vi "Translate to Array Data_3.vi"(0 "original data":path=path "C:/Users/User/Desktop/aaa.csv", 1 "Only Use Last Value?":bool=TRUE, 2 "Electrode number, N":u16=8, 3 "Current Mode":u8[][](array[numeric]), 5 "original error":errorcluster, 7 "Array Mode":u16(ring) items=["None", "Gradient + Dipole dipole", "Gradient", "Dipole Dipole", "Schlumberger"], 9 "modified data":path=path "C:/Users/User/Desktop/test.csv", 11 "modified error":errorcluster, 12 "Inverse\nPolarity":bool=TRUE, 13 "Insert\nBreak":bool=TRUE, 14 "External\nRef":bool=TRUE) -> (4 "original data path":path, 6 "original data error out":errorcluster)   [LabVIEW 2023]
uses:
  <vilib>/Utility/error.llb/DialogType.ctl
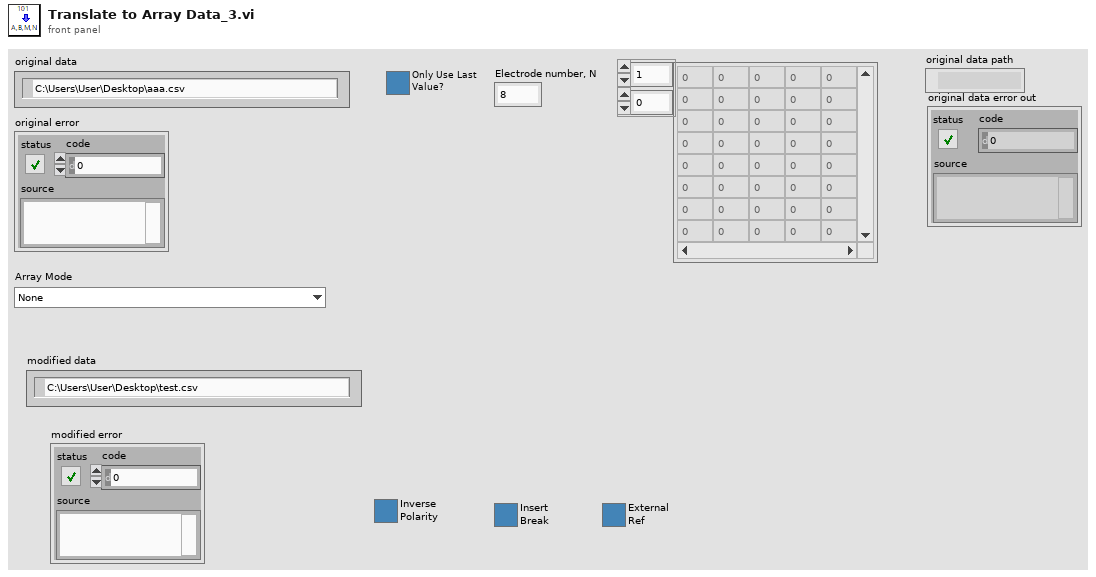
[diagram p1: front panel]
types:
  T1 = enum16{"open", "replace", "create", "open or create", "replace or create", "replace or create with confirmation"}
  T2 = typedef "DialogType.ctl" = u16
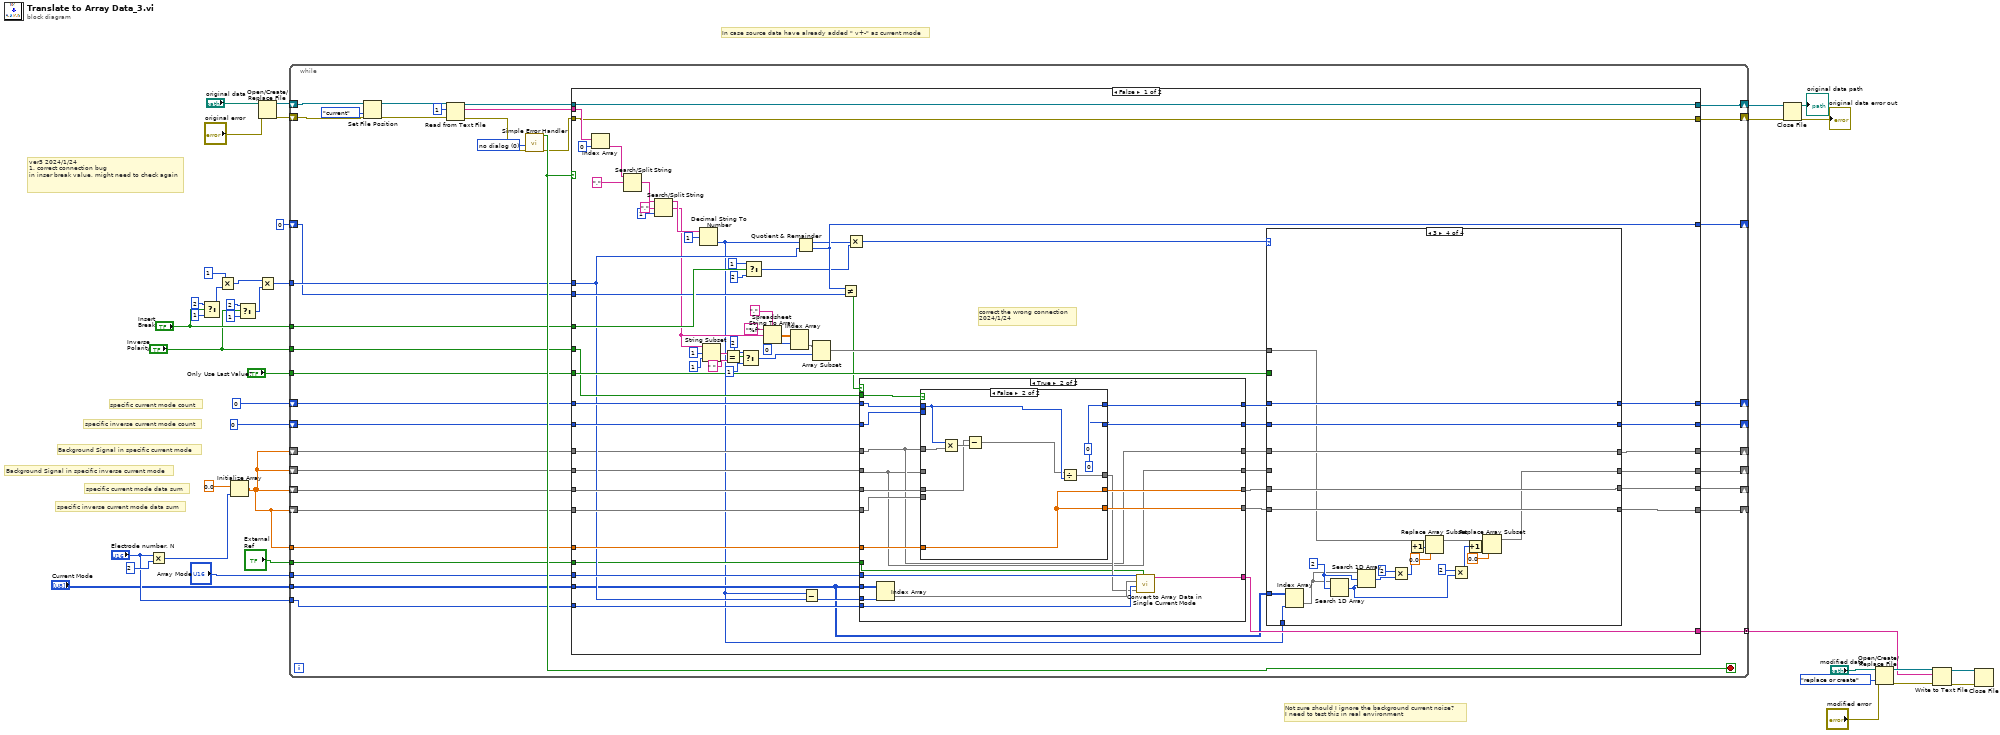
[diagram p0: block diagram]
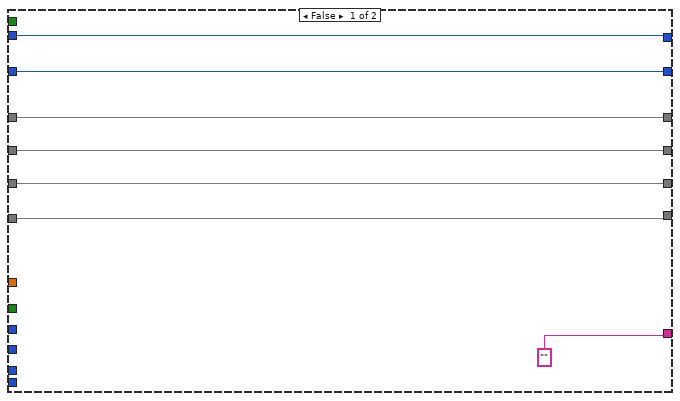
[diagram p2: hidden frame]
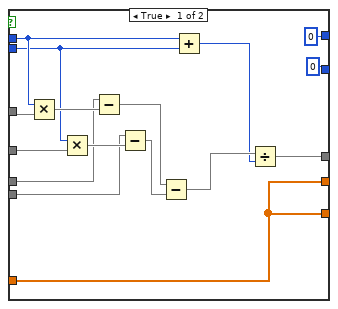
[diagram p3: hidden frame]
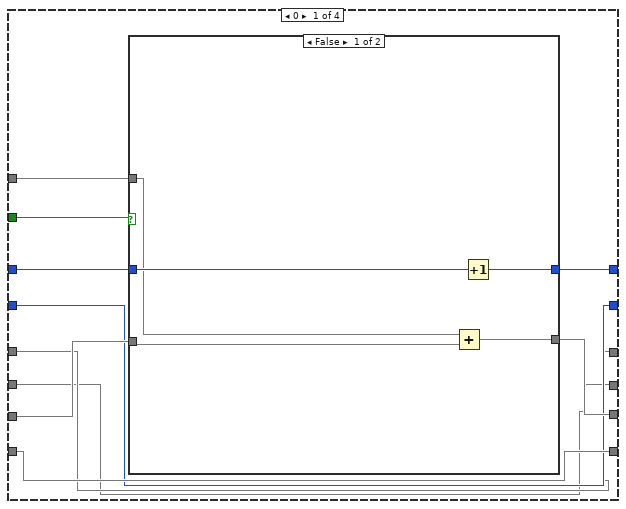
[diagram p4: hidden frame]
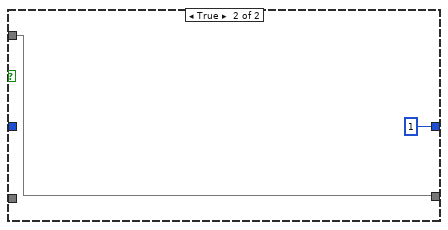
[diagram p5: hidden frame]
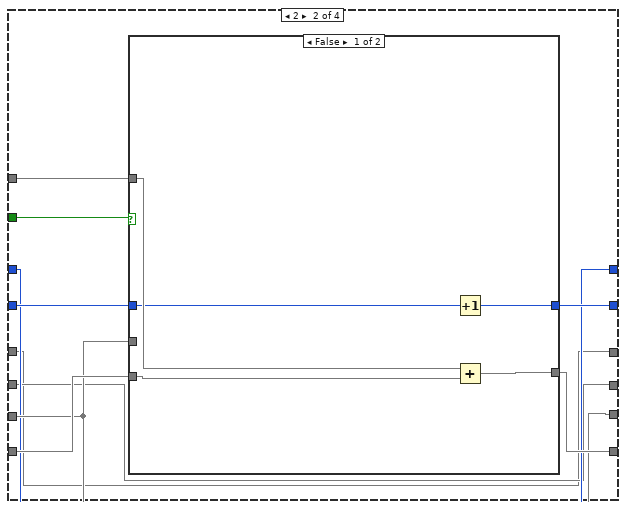
[diagram p6: hidden frame]
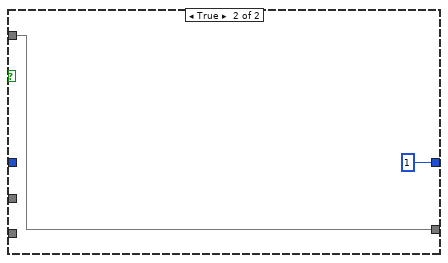
[diagram p7: hidden frame]
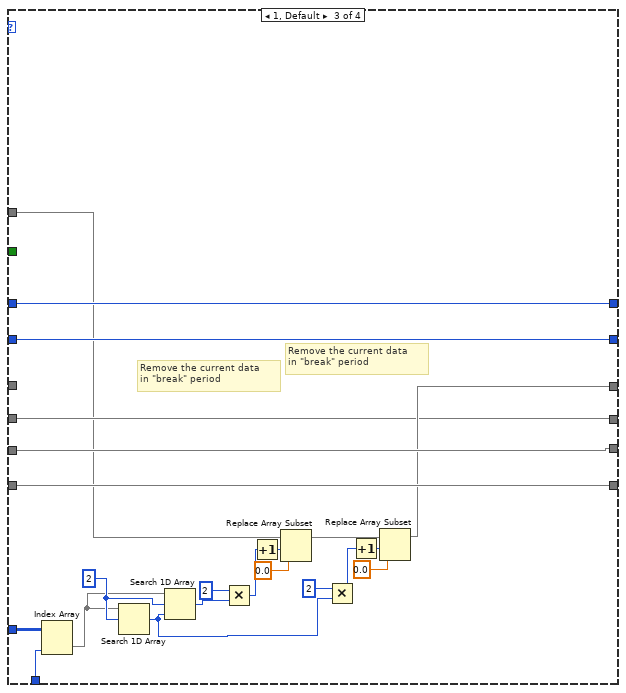
[diagram p8: hidden frame]
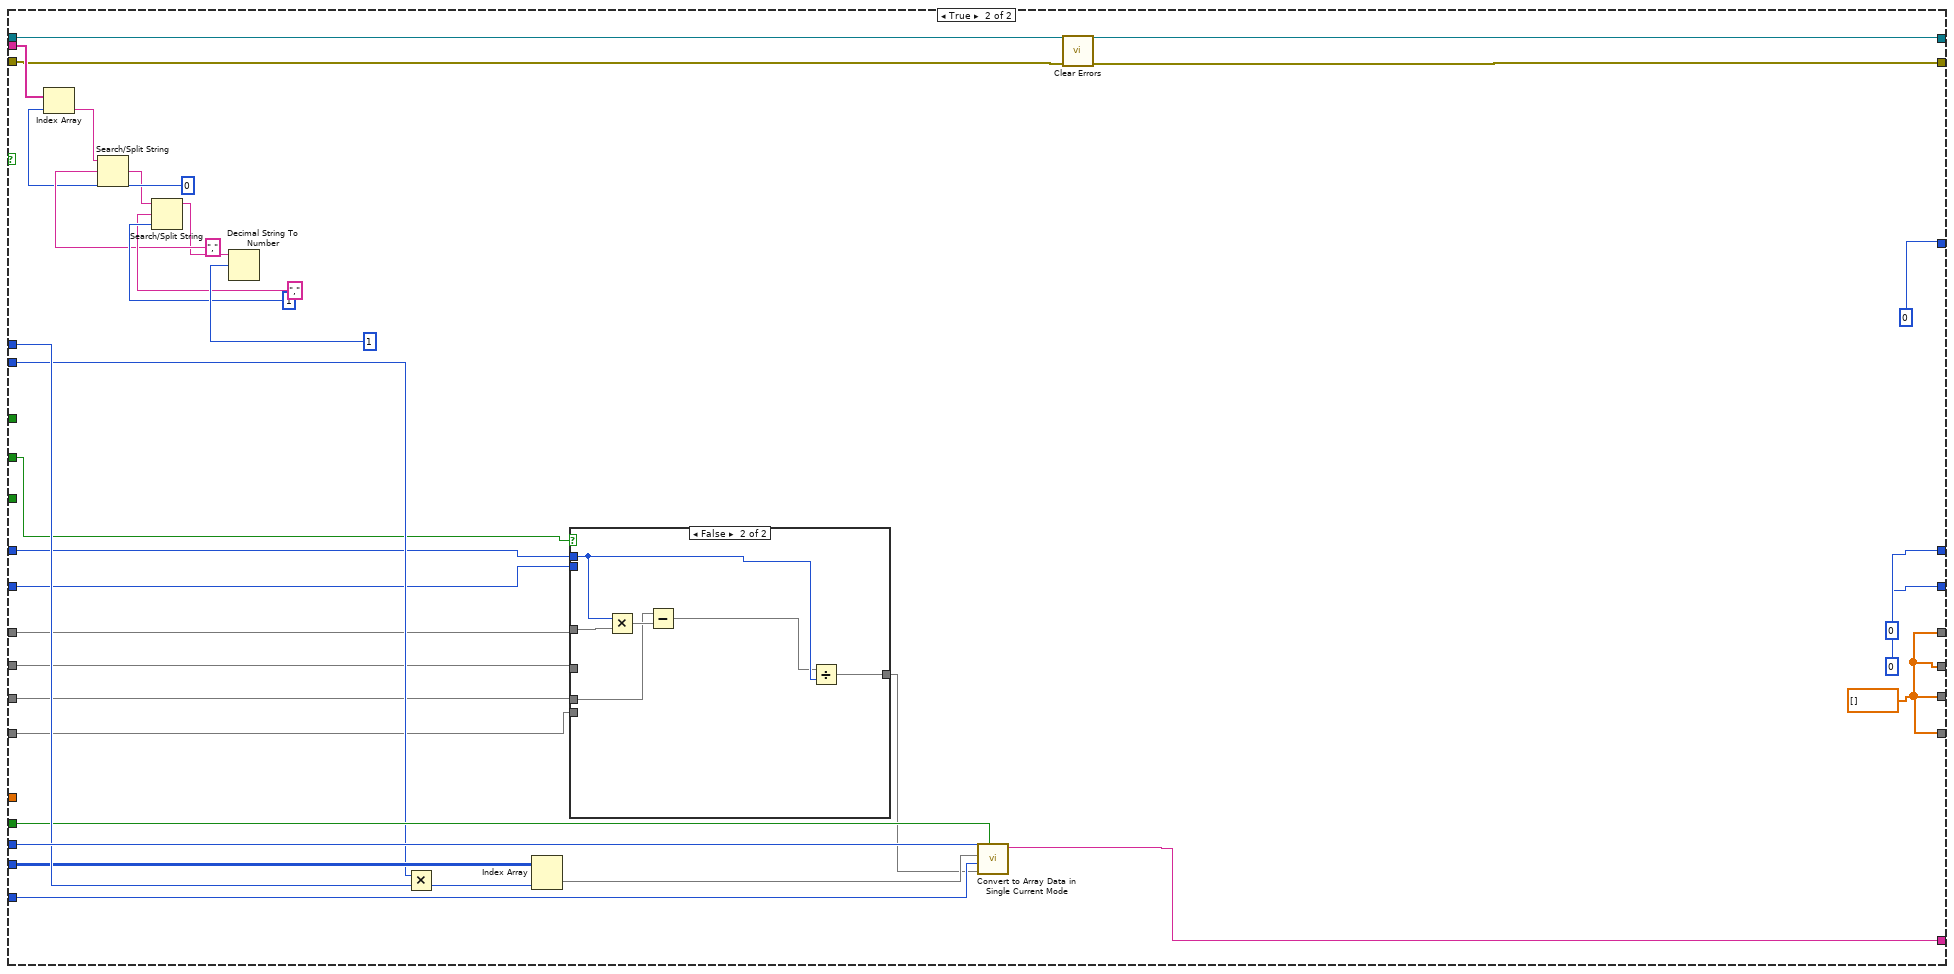
[diagram p9: hidden frame]
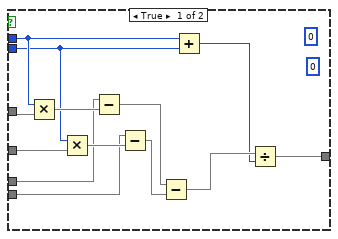
[diagram p10: hidden frame]
diagram:
  # "Not sure should I ignore the background current noise?\nI need to test this in real environment"
  # "ver3 2024/1/24\n1. correct connection bug\nin inser break value, might need to check again"
  # "Background Signal in specific inverse current mode"
  # "Background Signal in specific current mode"
  # "In case source data have already added \" v+-\" as current mode"
  # "specific inverse current mode data sum"
  # "specific current mode data sum"
  # "specific inverse current mode count"
  # "specific current mode count"
  n1 = Multiply(x="Electrode number, N", y=u16 2) -> (x*y=w13:u16)
  n2 = Select(t=2 ("number"), s="Insert\nBreak", f=1 ("number")) -> (s? t:f=w22:i32)
  n3 = Multiply(x=1 ("number"), y=w22) -> (x*y=w16:i32)
  n4 = Initialize Array(0.0 ("element"), w13) -> (w3:dbl[])
  n5 = Select(t=2 ("number"), s="Inverse\nPolarity", f=1 ("number")) -> (s? t:f=w21:i32)
  n6 = Open/Create/Replace File(file path (use dialog)="original data", error in="original error") -> (refnum out=w36:refnum<file>, error out=w37:errorcluster)  [unwired: 4 in, 1 out]
  n7 = Multiply(x=w16, y=w21) -> (x*y=w20:i32)
  n8 = while {
    shift-right: [w69] -> w31
    shift-left: w37 -> [w76]
    shift-right: [w68] -> w38
    shift-left: w36 -> [w67]
    tunnel: "Insert\nBreak" -> [w63]
    tunnel: "Inverse\nPolarity" -> [w62]
    tunnel: "Only Use Last Value?" -> [w61]
    tunnel: w20 -> [w60]
    shift-right: [w55] -> _
    shift-left: 0 ("number") -> [w59]
    shift-right: [w52] -> _
    shift-left: 0 ("number") -> [w58]
    shift-right: [w54] -> _
    shift-left: w3 -> [w57]
    shift-right: [w53] -> _
    shift-left: w3 -> [w56]
    shift-right: [w51] -> _
    shift-left: 0 -> [w50]
    tunnel: w3 -> [w49]
    tunnel: "Current Mode" -> [w47]
    tunnel: "Array Mode" -> [w48]
    tunnel: "Electrode number, N" -> [w46]
    tunnel: "External\nRef" -> [w45]
    tunnel: [w44] -> w7 mode=concatenating
    shift-right: [w41] -> _
    shift-left: w3 -> [w43]
    shift-right: [w40] -> _
    shift-left: w3 -> [w42]
    stop <- w73 stop-if-true
    w74 = T2 0 items=["no dialog", "OK message", "continue or stop message", "OK message + warnings", "continue/stop + warnings"] ("type of dialog (OK msg:1)")
    n9 = Set File Position(refnum=w67, from (0:start)=enum16{"start", "end", "current"}."current", error in=w76) -> (refnum out=w66:refnum<file>, error out=w65:errorcluster)  [unwired: 1 in]
    n10 = Read from Text File(file (use dialog)=w66, count=1, error in=w65) -> (refnum out=w71:refnum<file>, text=w72:string[], error out=w70:errorcluster)  [unwired: 1 in, 1 out]
    n11 = call <vilib>:"Simple Error Handler.vi"("type of dialog (OK msg:1)"=w74, "error in (no error)"=w70) -> ("error?"=w73:bool, "error out"=w64:errorcluster)  [unwired: 3 in, 3 out]
    n12 = case shown="False" w73 {
      tunnel: w72 -> [w137 w300]
      tunnel: w71 -> [w134 w297]
      tunnel: w64 -> [w133 w285]
      tunnel: [w134 w297] -> w68
      tunnel: [w133 w284] -> w69
      tunnel: w63 -> [w130 _]
      tunnel: w62 -> [w110 w275]
      tunnel: w61 -> [w129 _]
      tunnel: w60 -> [w98 w292]
      tunnel: w59 -> [w114 w274]
      tunnel: w58 -> [w113 w273]
      tunnel: w57 -> [w112 w278]
      tunnel: w56 -> [w111 w279]
      tunnel: [w120 0 ("number")] -> w55
      tunnel: [w119 w280] -> w54
      tunnel: [w118 w280] -> w53
      tunnel: [w117 0 ("number")] -> w52
      tunnel: [w115 0] -> w51
      tunnel: w50 -> [w116 w281]
      tunnel: w49 -> [w104 _]
      tunnel: w48 -> [w100 w294]
      tunnel: w47 -> [w81 w282]
      tunnel: w46 -> [w97 w291]
      tunnel: w45 -> [w96 w290]
      tunnel: [w95 w289] -> w44
      tunnel: w43 -> [w85 w276]
      tunnel: w42 -> [w84 w277]
      tunnel: [w79 w280] -> w41
      tunnel: [w78 w280] -> w40
      frame False {
        # "correct the wrong connection\n2024/1/24"
        n13 = Index Array(array=w137, index=0) -> (element=w135:string)
        n14 = Search/Split String(string=w135, search string/char (-)=",") -> (match + rest of string=w125:string)  [unwired: 1 in, 2 out]
        n15 = Search/Split String(string=w125, search string/char (-)=",", offset (0)=1) -> (substring before match=w126:string, match + rest of string=w87:string)  [unwired: 1 out]
        n16 = Decimal String To Number(string=w126, offset=1) -> (number=w80:i32)  [unwired: 1 in, 1 out]
        n17 = String Subset(string=w87, offset (0)=1, length (rest)=1 ("length (rest)")) -> (substring=w94:string)
        n18 = Equal?(x=w94, y=" ") -> (x = y?=w93:bool)
        n19 = Select(t=2 ("index (row)"), s=w93, f=1 ("index (row)")) -> (s? t:f=w86:i32)
        n20 = Select(t=1, s=w130, f=2 ("y")) -> (s? t:f=w103:i32)
        n21 = Spreadsheet String To Array(delimiter (Tab)=",", format string="%f", spreadsheet string=w87) -> (array=w124:dbl[][])  [unwired: 1 in]
        n22 = Index Array(array=w124, index (row)=0) -> (element=w122:dbl[])  [unwired: 1 in]
        n23 = Quotient & Remainder(x=w80, y=w98) -> (x-y*floor(x/y)=w102:i32, floor(x/y)=w115:i32)
        n24 = Subtract(x=w80, y=w98) -> (x-y=w99:i32)
        n25 = Array Subset(array=w122, index=w86) -> (w121:dbl[])  [unwired: 1 in]
        n26 = Not Equal?(x=w115, y=w116) -> (x != y?=w105:bool)
        n27 = Multiply(x=w102, y=w103) -> (x*y=w101:i32)
        n28 = case shown="True" w105 {
          tunnel: w114 -> [w148 w165]
          tunnel: w113 -> [w147 w164]
          tunnel: w112 -> [w146 w167]
          tunnel: w111 -> [w145 w166]
          tunnel: w110 -> [_ w168]
          tunnel: [w148 w163] -> w109
          tunnel: [w147 w162] -> w108
          tunnel: [w146 w161] -> w107
          tunnel: [w145 w160] -> w106
          tunnel: w104 -> [_ w159]
          tunnel: w100 -> [_ w155]
          tunnel: w81 -> [_ w158]
          tunnel: w99 -> [_ w157]
          tunnel: w97 -> [_ w154]
          tunnel: w96 -> [_ w152]
          tunnel: ["" ("String") w151] -> w95
          tunnel: w85 -> [w143 w150]
          tunnel: w84 -> [w142 w149]
          tunnel: [w143 w150] -> w83
          tunnel: [w142 w149] -> w82
          frame False {
          }
          frame True {
            n29 = Index Array(array=w158, index (col)=w157) -> (element=w156:u8[])  [unwired: 1 in]
            n30 = case shown="False" w168 {
              tunnel: w167 -> [w173 w186]
              tunnel: w166 -> [w172 _]
              tunnel: w165 -> [w174 w188]
              tunnel: w164 -> [w169 _]
              tunnel: [0 ("number") 0 ("number")] -> w163
              tunnel: [0 ("number") 0 ("number")] -> w162
              tunnel: [w180 w191] -> w161
              tunnel: [w180 w191] -> w160
              tunnel: w159 -> [w180 w191]
              tunnel: [w179 w190] -> w153
              tunnel: w150 -> [w177 w189]
              tunnel: w149 -> [w175 _]
              frame True {
                n31 = Multiply(x=w174, y=w177) -> (x*y=w178:dbl[])
                n32 = Multiply(x=w169, y=w175) -> (x*y=w176:dbl[])
                n33 = Subtract(x=w173, y=w178) -> (x-y=w170:dbl[])
                n34 = Subtract(x=w172, y=w176) -> (x-y=w171:dbl[])
                n35 = Subtract(x=w170, y=w171) -> (x-y=w184:dbl[])
                n36 = Add(x=w174, y=w169) -> (x+y=w183:i32)
                n37 = Divide(x=w184, y=w183) -> (x/y=w179:dbl[])
              }
              frame False {
                n38 = Multiply(x=w188, y=w189) -> (x*y=w187:dbl[])
                n39 = Subtract(x=w186, y=w187) -> (x-y=w185:dbl[])
                n40 = Divide(x=w185, y=w188) -> (x/y=w190:dbl[])
              }
            }
            n41 = call "Convert to Array Data in Single Current Mode.vi"("External\nRef"=w152, "data"=w153, "Electrode number, N"=w154, "Current Mode"=w156, "Array Mode"=w155) -> ("String"=w151:string)  [unwired: 6 in]
          }
        }
        n42 = case shown="3" w101 {
          tunnel: w129 -> [w203 w220 _ _]
          tunnel: w121 -> [w199 w219 w228 w250]
          tunnel: w109 -> [w202 w213 w249 w271]
          tunnel: w108 -> [w196 w216 w248 w270]
          tunnel: w107 -> [w201 w214 w247 w269]
          tunnel: w106 -> [w197 w218 w246 w268]
          tunnel: [w200 w213 w249 w271] -> w120
          tunnel: [w198 w214 w247 w269] -> w119
          tunnel: [w197 w217 w246 w268] -> w118
          tunnel: [w196 w215 w248 w270] -> w117
          tunnel: w83 -> [w195 w211 _ w251]
          tunnel: w82 -> [w194 w212 w229 _]
          tunnel: w81 -> [_ _ w243 w265]
          tunnel: w80 -> [_ _ w242 w264]
          tunnel: [w195 w211 w230 w251] -> w79
          tunnel: [w194 w212 w229 w252] -> w78
          frame 0 {
            n43 = case shown="False" w203 {
              tunnel: w202 -> [w208 _]
              tunnel: w201 -> [w205 _]
              tunnel: [w207 1 ("number")] -> w200
              tunnel: w199 -> [w204 w209]
              tunnel: [w206 w209] -> w198
              frame False {
                n44 = Add(x=w204, y=w205) -> (x+y=w206:dbl[])
                n45 = Increment(x=w208) -> (x+1=w207:i32)
              }
              frame True {
              }
            }
          }
          frame 2 {
            n46 = case shown="False" w220 {
              tunnel: w214 -> [_ _]
              tunnel: w219 -> [w224 w227]
              tunnel: [w225 w227] -> w217
              tunnel: w218 -> [w223 _]
              tunnel: w216 -> [w222 _]
              tunnel: [w221 1 ("number")] -> w215
              frame False {
                n47 = Increment(x=w222) -> (x+1=w221:i32)
                n48 = Add(x=w224, y=w223) -> (x+y=w225:dbl[])
              }
              frame True {
              }
            }
          }
          frame 1, Default {
            w245 = u8 2 ("element")
            # "Remove the current data\nin \"break\" period"
            # "Remove the current data\nin \"break\" period"
            n49 = Index Array(array=w243, index (col)=w242) -> (element=w244:u8[])  [unwired: 1 in]
            n50 = Search 1D Array(1D array=w244, element=w245) -> (index of element=w231:i32)  [unwired: 1 in]
            n51 = Search 1D Array(1D array=w244, element=w245, start index (0)=w231) -> (index of element=w241:i32)
            n52 = Multiply(x=2, y=w241) -> (x*y=w239:i32)
            n53 = Increment(x=w239) -> (x+1=w238:i32)
            n54 = Replace Array Subset(array=w228, new element=0.0 ("new element/subarray"), index=w238) -> (w234:dbl[])
            n55 = Multiply(x=2, y=w231) -> (x*y=w232:i32)
            n56 = Increment(x=w232) -> (x+1=w235:i32)
            n57 = Replace Array Subset(array=w234, new element=0.0 ("new element/subarray"), index=w235) -> (w230:dbl[])
          }
          frame 3 {
            w267 = u8 2 ("element")
            n58 = Index Array(array=w265, index (col)=w264) -> (element=w266:u8[])  [unwired: 1 in]
            n59 = Search 1D Array(1D array=w266, element=w267) -> (index of element=w253:i32)  [unwired: 1 in]
            n60 = Search 1D Array(1D array=w266, element=w267, start index (0)=w253) -> (index of element=w263:i32)
            n61 = Multiply(x=2, y=w263) -> (x*y=w261:i32)
            n62 = Increment(x=w261) -> (x+1=w260:i32)
            n63 = Replace Array Subset(array=w250, new element=0.0 ("new element/subarray"), index=w260) -> (w256:dbl[])
            n64 = Multiply(x=2, y=w253) -> (x*y=w254:i32)
            n65 = Increment(x=w254) -> (x+1=w257:i32)
            n66 = Replace Array Subset(array=w256, new element=0.0 ("new element/subarray"), index=w257) -> (w252:dbl[])
          }
        }
      }
      frame True {
        w280 = dbl[] [] ("subarray")
        n67 = Index Array(array=w300, index=0) -> (element=w298:string)
        n68 = Search/Split String(string=w298, search string/char (-)=",") -> (match + rest of string=w295:string)  [unwired: 1 in, 2 out]
        n69 = Search/Split String(string=w295, search string/char (-)=",", offset (0)=1) -> (substring before match=w296:string)  [unwired: 2 out]
        n70 = Decimal String To Number(string=w296, offset=1) -> ()  [unwired: 1 in, 2 out]
        n71 = Multiply(x=w281, y=w292) -> (x*y=w293:i32)
        n72 = Index Array(array=w282, index (col)=w293) -> (element=w283:u8[])  [unwired: 1 in]
        n73 = case shown="False" w275 {
          tunnel: w278 -> [w309 w319]
          tunnel: w279 -> [w308 _]
          tunnel: w274 -> [w310 w321]
          tunnel: w273 -> [w305 _]
          tunnel: [w315 w323] -> w272
          tunnel: w276 -> [w313 w322]
          tunnel: w277 -> [w311 _]
          frame True {
            (unwired) 0 ("number")
            (unwired) 0 ("number")
            n74 = Multiply(x=w310, y=w313) -> (x*y=w314:dbl[])
            n75 = Multiply(x=w305, y=w311) -> (x*y=w312:dbl[])
            n76 = Subtract(x=w309, y=w314) -> (x-y=w306:dbl[])
            n77 = Subtract(x=w308, y=w312) -> (x-y=w307:dbl[])
            n78 = Subtract(x=w306, y=w307) -> (x-y=w317:dbl[])
            n79 = Add(x=w310, y=w305) -> (x+y=w316:i32)
            n80 = Divide(x=w317, y=w316) -> (x/y=w315:dbl[])
          }
          frame False {
            n81 = Multiply(x=w321, y=w322) -> (x*y=w320:dbl[])
            n82 = Subtract(x=w319, y=w320) -> (x-y=w318:dbl[])
            n83 = Divide(x=w318, y=w321) -> (x/y=w323:dbl[])
          }
        }
        n84 = call "Convert to Array Data in Single Current Mode.vi"("External\nRef"=w290, "data"=w272, "Electrode number, N"=w291, "Current Mode"=w283, "Array Mode"=w294) -> ("String"=w289:string)  [unwired: 6 in]
        n85 = call <vilib>:"Clear Errors.vi"("error in (no error)"=w285) -> ("error out"=w284:errorcluster)  [unwired: 5 in, 1 out]
      }
    }
  }
  n86 = Close File(refnum=w38, error in=w31) -> (path=→"original data path":path, error out=→"original data error out":errorcluster)
  n87 = Open/Create/Replace File(file path (use dialog)="modified data", error in="modified error", operation (0:open)=T1."replace or create") -> (refnum out=w9:refnum<file>, error out=w8:errorcluster)  [unwired: 3 in, 1 out]
  n88 = Write to Text File(file (use dialog)=w9, text=w7, error in=w8) -> (refnum out=w6:refnum<file>, error out=w5:errorcluster)  [unwired: 1 in, 1 out]
  n89 = Close File(refnum=w6, error in=w5) -> ()  [unwired: 2 out]
